vi "BL_StartChannels.vi"(8 "error in (no error)":errorcluster, 10 "Channles":u8[](array[numeric]), 11 "Potentiostat Galvanostat in":refnum<class "Potentiostat Galvanostat.lvclass">) -> (0 "error out":errorcluster, 1 "Channel Error Codes":i32[](array[numeric]), 2 "Channels":u8[](array[numeric]), 3 "Potentiostat Galvanostat out":refnum<class "Potentiostat Galvanostat.lvclass">)   [LabVIEW 2018, in "Potentiostat Galvanostat.lvclass"]
doc: "The hardware conf object. The attribute “Conn” is the electrode\nconnection mode and the attribute “Ground” is the instrument\nground. See 5. Structures and Constants to have the value of these\nattributes."
uses:
  Potentiostat Galvanostat.lvclass
  Potentiostat Galvanostat.lvclass/Potentiostat Galvanostat.ctl
  BL_GetErrorMsg.vi
  <vilib>/Utility/error.llb/Error Cluster From Error Code.vi
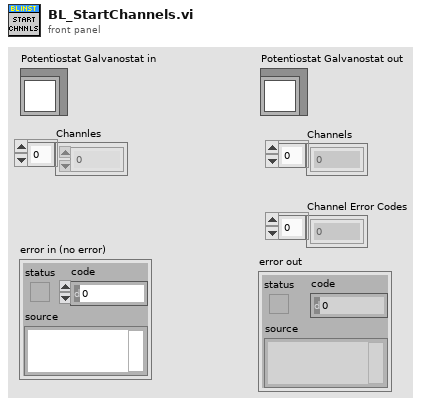
[diagram p1: front panel]
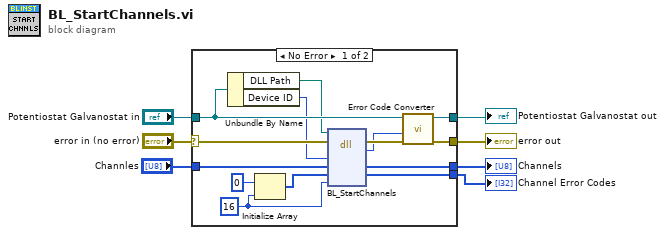
[diagram p0: block diagram]
diagram:
  n1 = case shown="No Error" "error in (no error)" {
    selector: "error in (no error)" -> [w17 w23]
    tunnel: [w21 w23] -> w6
    tunnel: [w20 w22] -> w4
    tunnel: "Potentiostat Galvanostat in" -> [w19 w22]
    tunnel: "Channles" -> [w11 _]
    tunnel: [w13 _] -> w2
    tunnel: [w12 _] -> w1
    frame No Error {
      w8 = 16 ("dimension size")
      n2 = Unbundle By Name(w19) -> ("DLL Path"=w16:path, "Device ID"=w15:i32)
      n3 = Initialize Array(0 ("element"), w8) -> (w9:i32[])
      n4 = dll-call lib="C:/Program Files (x86)/National Instruments/LabVIEW 2018/user.lib/EClib/EClib.*" fn="BL_StartChannels"(path in=w16, error in=w17, "Device ID"=w15, "Channels"=w11, "Channel Error Codes"=w9, "Size"=w8) -> (error out=w18:errorcluster, "Error Code"=w14:i32, "Channels"=w13:u8[], "Channel Error Codes"=w12:i32[])  [unwired: 3 in, 1 out]
      n5 = call "Error Code Converter.vi"("error in (no error)"=w18, "Error Code"=w14, "Potentiostat Galvanostat in"=w19) -> ("error out"=w21:errorcluster, "Potentiostat Galvanostat out"=w20:refnum<class "Potentiostat Galvanostat.lvclass">)  [unwired: 7 in]
    }
    frame Error {
    }
  }
  "error out" <- w6
  "Potentiostat Galvanostat out" <- w4
  "Channels" <- w2
  "Channel Error Codes" <- w1
